vi "switch.vi"() -> ()   [LabVIEW 2015]
panel:
  out "Commands":string
  in  "Channel to close":i16
  out "VISA resource name out":refnum<visa-resource-name>
  out "return count":u32
  out "error out":errorcluster
  in  "error in (no error)":errorcluster
  in  "VISA resource name":refnum<visa-resource-name>
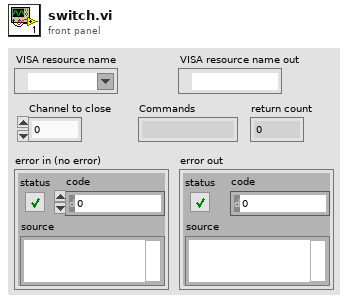
[diagram p1: front panel]
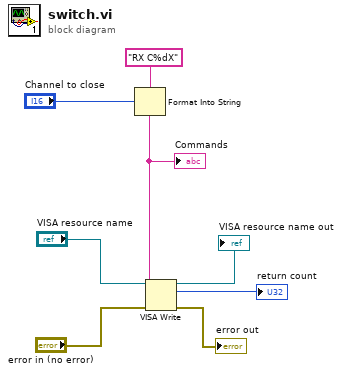
[diagram p0: block diagram]
diagram:
  n1 = Format Into String(format string="RX C%dX" ("initial string"), "Channel to close") -> (resulting string=w2:string)  [unwired: 2 in, 1 out]
  "Commands" <- w2
  n2 = VISA Write(VISA resource name="VISA resource name", write buffer=w2, error in (no error)="error in (no error)") -> (VISA resource name out=→"VISA resource name out":refnum<visa-resource-name>, return count=→"return count":u32, error out=→"error out":errorcluster)
